vi "Day 22-Sum Volumes.vi"(11 "Map":map{i64[], i64}(c390)) -> (3 "Volumn \"On\"":i64)   [LabVIEW 2021]
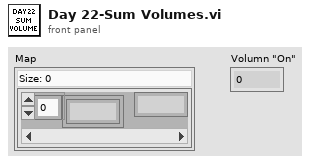
[diagram p1: front panel]
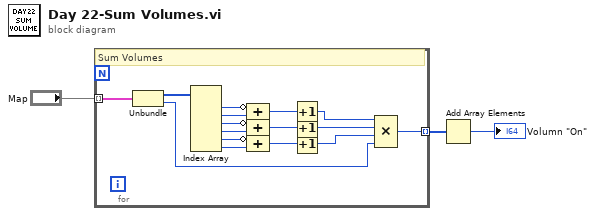
[diagram p0: block diagram]
diagram:
  n1 = for {
    tunnel: [w7] -> w1 mode=indexing
    tunnel: "Map" -> [w6] mode=indexing
    # "Sum Volumes"
    n2 = Unbundle(w6) -> (w5:i64[], w4:i64)
    n3 = Index Array(array=w5) -> (element #1=w19:i64, element #2=w18:i64, element #3=w17:i64, element #4=w16:i64, element #5=w15:i64, element #6=w14:i64)  [unwired: 6 in]
    n4 = Compound Arithmetic op=ADD(invert w19, w18) -> (w13:i64)
    n5 = Compound Arithmetic op=ADD(invert w17, w16) -> (w12:i64)
    n6 = Compound Arithmetic op=ADD(invert w15, w14) -> (w11:i64)
    n7 = Increment(x=w13) -> (x+1=w9:i64)
    n8 = Increment(x=w12) -> (x+1=w10:i64)
    n9 = Increment(x=w11) -> (x+1=w8:i64)
    n10 = Compound Arithmetic op=MULTIPLY(w9, w10, w8, w4) -> (w7:i64)
  }
  n11 = Add Array Elements(numeric array=w1) -> (sum=→"Volumn \"On\"":i64)
